vi "Base64_DecodeAnything.vi"(7 "Type (Adapt)":variant, 8 "error in (no error)":errorcluster, 10 "Encoded Payload":string) -> (0 "error out":errorcluster, 2 "Variant":variant)   [LabVIEW 2019, in "OpenSerializer.base64.lvlib"]
uses:
  Serializer.Base64.lvclass
  C:/Program Files (x86)/National Instruments/LabVIEW 2019/vi.lib/LabVIEW Open Source Project/OpenSerializer/Serializer/Serializer.lvclass
  OpenSerializer.base64.lvlib
  <vilib>/LabVIEW Open Source Project/OpenSerializer/Serializer/Serializer.lvclass
  C:/Program Files (x86)/National Instruments/LabVIEW 2019/vi.lib/LabVIEW Open Source Project/OpenSerializer/Serializer.FlattenedString/Serializer.FlattenedString.lvclass
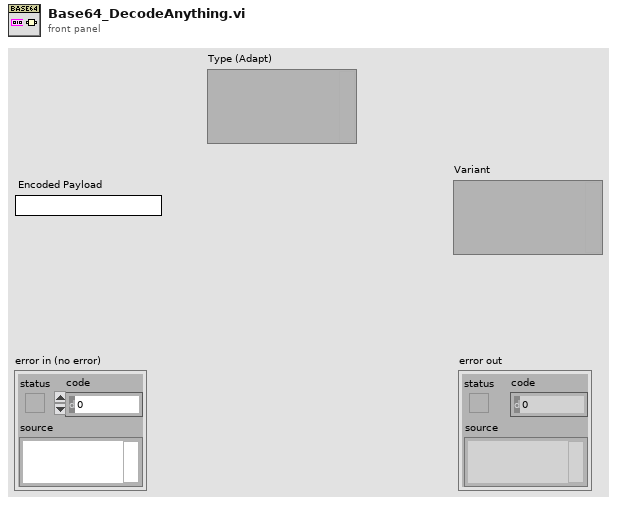
[diagram p1: front panel]
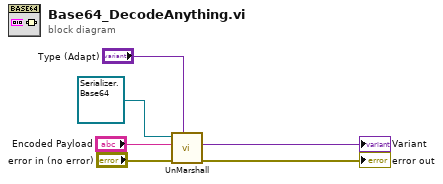
[diagram p0: block diagram]
diagram:
  n1 = call <vilib>:"UnMarshall.vi"("Type"="Type (Adapt)", "error in (no error)"="error in (no error)", "String"="Encoded Payload", "Serializer in"=refnum<class "Serializer.Base64.lvclass"> refnum ("Serializer.Base64 in")) -> ("error out"=→"error out":errorcluster, "Variant"=→"Variant":variant)  [unwired: 5 in, 1 out]
